vi "Begin Motors V.5.0.vi"   [LabVIEW 2016]
uses:
  <vilib>/Rock Robotics/WPI/ThirdParty/CanMotor/TalonSRX/WPI_CANTalonSRX_APIFeedbackSelect.ctl
  <vilib>/Rock Robotics/WPI/ThirdParty/CanMotor/TalonSRX/WPI_CANTalonSRX_StatusFrame.ctl
  <vilib>/Rock Robotics/SystemInterfaces/DIO/FPGA_DIOPWMChannel.ctl
  <vilib>/Rock Robotics/WPI/SafetyOutput/WPI_SafetyOutputConfigMenu.ctl
  Robot Global Data V.5.0.vi
  <vilib>/Rock Robotics/WPI/RobotDrive/WPI_RobotDriveOpen4MotorWithExistingMotors.vi
  <vilib>/Rock Robotics/WPI/MotorControl/WPI_MotorControlOpen VictorSP.vi
types:
  T1 = typedef "WPI_SafetyOutputConfigMenu.ctl" = enum16{"Enable", "Disable"}
  T2 = typedef "FPGA_DIOPWMChannel.ctl" = enum8{"PWM 0", "PWM 1", "PWM 2", "PWM 3", "PWM 4", "PWM 5", "PWM 6", "PWM 7", "PWM 8", "PWM 9", "PWM MXP 0", "PWM MXP 1", "PWM MXP 2", "PWM MXP 3", "PWM MXP 4", "PWM MXP 5", "PWM MXP 6", "PWM MXP 7", "PWM MXP 8", "PWM MXP 9", "Invalid"}
  T3 = typedef "WPI_CANTalonSRX_StatusFrame.ctl" = enum16{"General Status Frame", "Feedback Status Frame", "Quadrature Status Frame", "Analog Temp Vbat Status Frame", "Pulse Width Status Frame"}
  T4 = typedef "WPI_CANTalonSRX_APIFeedbackSelect.ctl" = enum16{"Digital Quadrature Encoder", "Analog Potentiometer", "Analog Encoder", "Count on Quad-A (Rising-Edge)", "Count on Quad-A (Falling-Edge)", "CTR Magnetic Enc (Absolute)", "CTR Magnetic Enc (Relative)", "Pulse Width"}
  T5 = typedef "WPI_MotorControlDeviceRef.ctl" = cluster{"DeviceStatus":errorcluster, "Type":T6, "PWM":cluster{"PWM Channel":T2, "DeadBand":T7}, "CAN":cluster{"Device Number":u8, "SetOutput VI Ref":variant, "GetOutput VI Ref":variant, "Enable VI Ref":variant, "Disable VI Ref":variant, "Data":variant}, "Invert":bool}
  T6 = typedef "WPI_MotorControlType.ctl" = enum16{"PWM", "CAN"}
  T7 = typedef "WPI_PWMDeadband.ctl" = cluster{"Name":string, "maxPositivePwm":i32, "minPositivePwm":i32, "centerPwm":i32, "maxNegativePwm":i32, "minNegativePwm":i32, "angularRange":u16}
  T8 = typedef "WPI_RobotDriveDevRef.ctl" = cluster{"DevStatus":errorcluster, "Motors[]":T5[], "Square Inputs":bool, "Max Output":dbl}
  T9 = typedef "WPI_CANTalonSRX_GlobalStatus.ctl" = cluster{"Applied Throttle":dbl, "Module Enabled":bool, "CAN Error":errorcluster, "Closed Loop Error":dbl, "Forward Limit Switch Closed":bool, "Reverse Limit Switch Closed":bool, "Sensor Position":dbl, "Sensor Velocity":dbl, "Current":dbl, "Sticky Fault - Over Temp":bool, "Sticky Fault - Under Voltage":bool, "Sticky Fault - Forward Limit":bool, "Sticky Fault - Reverse Limit":bool, "Sticky Fault - Forward Soft Limit":bool, "Sticky Fault - Reverse Soft Limit":bool, "Brake is Enabled":bool, "Encoder Position":dbl, "Encoder Velocity":dbl, "Encoder Index Count":dbl, "Encoder A Pin State":bool, "Encoder B Pin State":bool, "Encoder Index Pin State":bool, "Analog In":dbl, "Analog In Velocity":dbl, "Temperature (C)":dbl, "Battery Voltage":dbl, "Control 5 Is Supported":bool, "Current Profile Slot Select":dbl, "Pos Div 8":bool, "Vel Div 4":bool, "Pulse Width Position":i32, "Pulse Width Velocity":i32, "Pulse Width Rise To Rise (us)":i32, "Pulse Width Rise To Fall (us)":i32, "Mot Prof Active Is Under Run":bool, "Mot Prof Active Has Under Run":bool, "Mot Prof Active Is Last":bool, "Mot Prof Active Velocity Only":bool, "Mot Prof Active Is Valid":bool, "Mot Prof Buffer Is Full":bool, "Mot Prof Active Profile Slot Select":i32, "Mot Prof NextID":i32, "Mot Prof Count":i32, "Mot Prof Active Velocity":dbl, "Mot Prof Active Position":dbl, "Mot Prof Output Enable":i32}
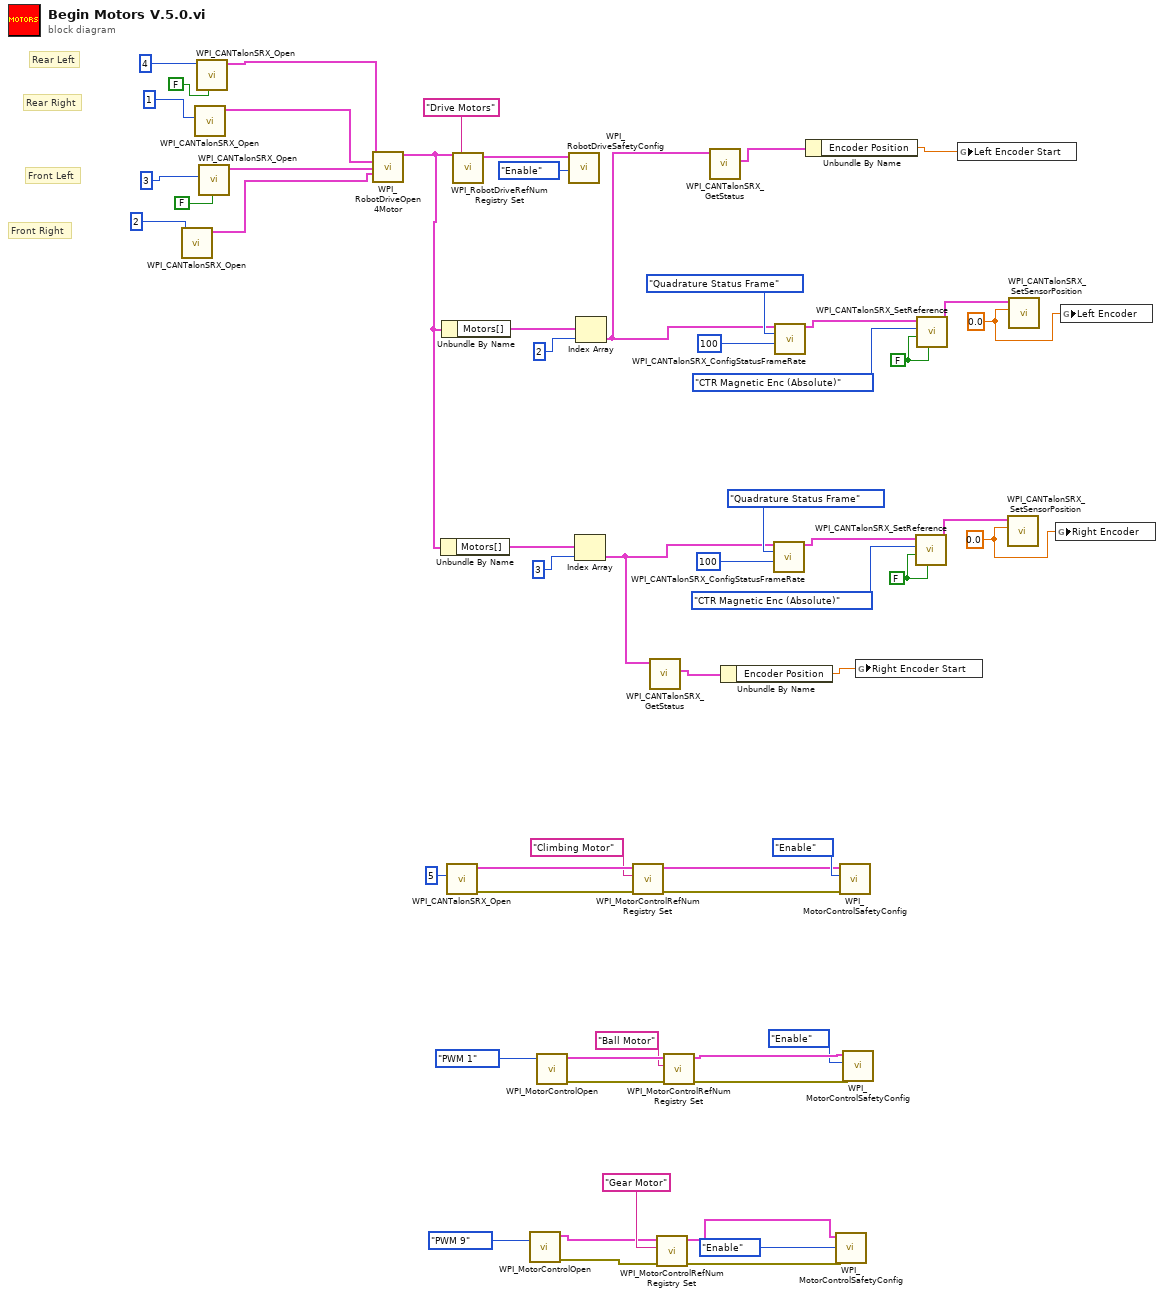
[diagram p0: block diagram]
diagram:
  w39 = 0.0
  w34 = FALSE
  w46 = 0.0
  w51 = FALSE
  # "Front Right"
  # "Front Left"
  # "Rear Right"
  # "Rear Left"
  n1 = call <vilib>:"WPI_CANTalonSRX_Open.vi"("Device Number"=2) -> ("CAN Talon SRX Ref"=w40:T5)  [unwired: 9 in, 1 out]
  n2 = call <vilib>:"WPI_CANTalonSRX_Open.vi"("Device Number"=1) -> ("CAN Talon SRX Ref"=w42:T5)  [unwired: 9 in, 1 out]
  n3 = call <vilib>:"WPI_CANTalonSRX_Open.vi"("Invert"=FALSE, "Device Number"=4) -> ("CAN Talon SRX Ref"=w43:T5)  [unwired: 8 in, 1 out]
  n4 = call <vilib>:"WPI_CANTalonSRX_Open.vi"("Invert"=FALSE, "Device Number"=3) -> ("CAN Talon SRX Ref"=w41:T5)  [unwired: 8 in, 1 out]
  n5 = call-poly <vilib>:"WPI_RobotDriveOpen4Motor.vi"("Rear Left Motor Dev Ref"=w43, "Rear Right Motor Dev Ref"=w42, "Front Left Motor Dev Ref"=w41, "Front Right Motor Dev Ref"=w40) -> ("RobotDriveDevRef"=w30:T8)  [unwired: 10 in, 1 out]
  n6 = Unbundle By Name(w30) -> ("Motors[]"=w31:T5[])
  n7 = Unbundle By Name(w30) -> ("Motors[]"=w54:T5[])
  n8 = call <vilib>:"WPI_CANTalonSRX_Open.vi"("Device Number"=u8 5) -> ("error out"=w2:errorcluster, "CAN Talon SRX Ref"=w7:T5)  [unwired: 9 in]
  n9 = call <vilib>:"WPI_RobotDriveRefNum Registry Set.vi"("refnum name"="Drive Motors", "RobotDriveDevRef"=w30) -> ("RobotDriveDevRef"=w57:T8)  [unwired: 2 in, 7 out]
  n10 = call-poly <vilib>:"WPI_MotorControlOpen.vi"("PWM Channel"=FPGA_DIOPWMChannel."PWM 9") -> ("error out"=w12:errorcluster, "MotorControlDeviceRef"=w9:T5)  [unwired: 9 in]
  n11 = call-poly <vilib>:"WPI_MotorControlOpen.vi"("PWM Channel"=FPGA_DIOPWMChannel."PWM 1") -> ("error out"=w23:errorcluster, "MotorControlDeviceRef"=w26:T5)  [unwired: 9 in]
  n12 = call <vilib>:"WPI_RobotDriveSafetyConfig.vi"("mode"=WPI_SafetyOutputConfigMenu."Enable", "RobotDriveDevRef"=w57) -> ()  [unwired: 8 in, 2 out]
  n13 = Index Array(array=w31, index=3) -> (element=w20:T5)
  n14 = Index Array(array=w54, index=2) -> (element=w17:T5)
  n15 = call <vilib>:"WPI_MotorControlRefNum Registry Set.vi"("error in (no error)"=w2, "refnum name"="Climbing Motor", "MotorControlDevRef"=w7) -> ("error out"=w3:errorcluster, "MotorControlDevRef"=w4:T5)  [unwired: 7 in]
  n16 = call <vilib>:"WPI_CANTalonSRX_GetStatus.vi"("CAN Talon SRX Ref"=w20) -> ("Talon SRX Status"=w19:T9)  [unwired: 8 in, 2 out]
  n17 = call <vilib>:"WPI_MotorControlRefNum Registry Set.vi"("error in (no error)"=w12, "refnum name"="Gear Motor", "MotorControlDevRef"=w9) -> ("error out"=w13:errorcluster, "MotorControlDevRef"=w11:T5)  [unwired: 7 in]
  n18 = call <vilib>:"WPI_MotorControlRefNum Registry Set.vi"("error in (no error)"=w23, "refnum name"="Ball Motor", "MotorControlDevRef"=w26) -> ("error out"=w22:errorcluster, "MotorControlDevRef"=w24:T5)  [unwired: 7 in]
  n19 = call <vilib>:"WPI_CANTalonSRX_GetStatus.vi"("CAN Talon SRX Ref"=w17) -> ("Talon SRX Status"=w16:T9)  [unwired: 8 in, 2 out]
  n20 = Unbundle By Name(w19) -> ("Encoder Position"=w18:dbl)
  n21 = call <vilib>:"WPI_CANTalonSRX_ConfigStatusFrameRate.vi"("CAN Talon SRX Ref"=w20, "Talon SRX Status Frame"=WPI_CANTalonSRX_StatusFrame."Quadrature Status Frame", "Frame Rate Ms"=100) -> ("CAN Talon SRX Ref"=w36:T5)  [unwired: 12 in]
  n22 = call <vilib>:"WPI_CANTalonSRX_ConfigStatusFrameRate.vi"("CAN Talon SRX Ref"=w17, "Talon SRX Status Frame"=WPI_CANTalonSRX_StatusFrame."Quadrature Status Frame", "Frame Rate Ms"=100) -> ("CAN Talon SRX Ref"=w49:T5)  [unwired: 12 in]
  n23 = Unbundle By Name(w16) -> ("Encoder Position"=w15:dbl)
  n24 = call <vilib>:"WPI_MotorControlSafetyConfig.vi"("error in (no error)"=w13, "mode"=WPI_SafetyOutputConfigMenu."Enable", "MotorControlDevRef"=w11) -> ()  [unwired: 7 in, 2 out]
  n25 = call <vilib>:"WPI_MotorControlSafetyConfig.vi"("error in (no error)"=w3, "mode"=WPI_SafetyOutputConfigMenu."Enable", "MotorControlDevRef"=w4) -> ()  [unwired: 7 in, 2 out]
  n26 = call <vilib>:"WPI_MotorControlSafetyConfig.vi"("error in (no error)"=w22, "mode"=WPI_SafetyOutputConfigMenu."Enable", "MotorControlDevRef"=w24) -> ()  [unwired: 7 in, 2 out]
  n27 = global write "Robot Global Data V.5.0.vi" "Right Encoder Start"(w18) -> ()
  n28 = call <vilib>:"WPI_CANTalonSRX_SetReference.vi"("Reverse Closed-Loop Output"=w34, "Reverse Feedback Sensor"=w34, "Feedback Reference"=WPI_CANTalonSRX_APIFeedbackSelect."CTR Magnetic Enc (Absolute)", "CAN Talon SRX Ref"=w36) -> ("CAN Talon SRX Ref"=w38:T5)  [unwired: 6 in, 1 out]
  n29 = call <vilib>:"WPI_CANTalonSRX_SetReference.vi"("Reverse Closed-Loop Output"=w51, "Reverse Feedback Sensor"=w51, "Feedback Reference"=WPI_CANTalonSRX_APIFeedbackSelect."CTR Magnetic Enc (Absolute)", "CAN Talon SRX Ref"=w49) -> ("CAN Talon SRX Ref"=w47:T5)  [unwired: 6 in, 1 out]
  n30 = global write "Robot Global Data V.5.0.vi" "Left Encoder Start"(w15) -> ()
  n31 = call <vilib>:"WPI_CANTalonSRX_SetSensorPosition.vi"("New Sensor Position"=w39, "CAN Talon SRX Ref"=w38) -> ()  [unwired: 8 in, 2 out]
  n32 = call <vilib>:"WPI_CANTalonSRX_SetSensorPosition.vi"("New Sensor Position"=w46, "CAN Talon SRX Ref"=w47) -> ()  [unwired: 8 in, 2 out]
  n33 = global write "Robot Global Data V.5.0.vi" "Right Encoder"(w39) -> ()
  n34 = global write "Robot Global Data V.5.0.vi" "Left Encoder"(w46) -> ()
